vi "OpenRTMMenu.vi"(8 "error in":errorcluster, 11 "RTMFilePath":path) -> (0 "error out":errorcluster, 2 "RTMMenuReference":refnum<k9>, 3 "RTMVIReference":refnum<vi>)   [LabVIEW 2021, in "Menu.lvlib" / "Menu.lvclass"]
uses:
  Menu.lvclass
  GetRTMMenuReference.vi
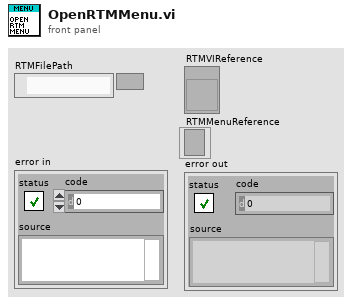
[diagram p1: front panel]
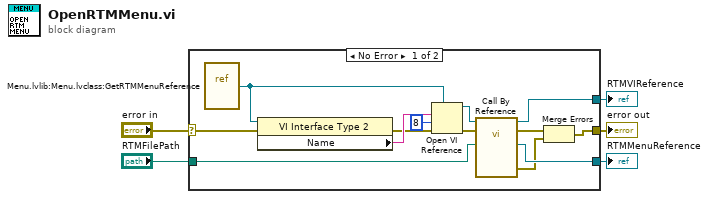
[diagram p0: block diagram]
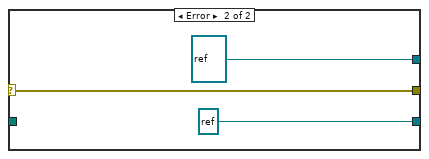
[diagram p2: hidden frame]
diagram:
  n1 = case shown="No Error" "error in" {
    selector: "error in" -> [w14 w20]
    tunnel: [w10 refnum<k9> refnum ("menu reference")] -> w5
    tunnel: [w18 w20] -> w4
    tunnel: "RTMFilePath" -> [w6 _]
    tunnel: [w12 refnum<vi> refnum] -> w1
    frame No Error {
      n2 = vi-ref "Menu.lvlib:Menu.lvclass:GetRTMMenuReference.vi"() -> (w8:refnum<vi>)
      n3 = property class="VI Interface Type 2"(reference=w8, error in=w14) -> (error out=w15:errorcluster, "Name"=w17:string)  [unwired: 1 out]
      n4 = Open VI Reference(type specifier VI Refnum (for type only)=w8, vi path=w17, options=8, error in (no error)=w15) -> (vi reference=w7:refnum<vi>, error out=w13:errorcluster)  [unwired: 2 out]
      n5 = call-by-ref "?"(reference=w7, error in=w13, "RTMFilePath"=w6) -> (reference out=w12:refnum<vi>, error out=w11:errorcluster, 0:"error out"=w9:errorcluster, "RTMMenuReference"=w10:refnum<k9>)  [unwired: 9 in]
      n6 = Merge Errors(w11, w9) -> (w18:errorcluster)
    }
    frame Error {
    }
  }
  "RTMMenuReference" <- w5
  "error out" <- w4
  "RTMVIReference" <- w1
